vi "old code for w-on-b or b-on-w detection.vi"(9 "Numeric 2":i32, 10 "Numeric":i32, 11 "Array":sgl[](array[numeric])) -> (3 "subarray":sgl[](array[numeric]))   [LabVIEW 2011]
uses:
  <vilib>/Analysis/NI_AALBase.lvlib
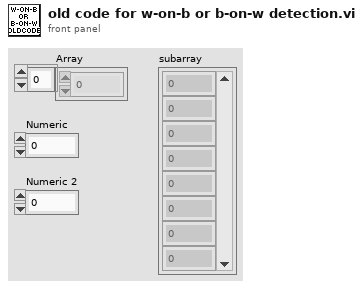
[diagram p1: front panel]
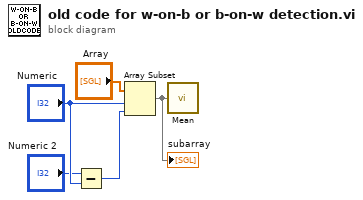
[diagram p0: block diagram]
diagram:
  n1 = Subtract(x="Numeric 2", y="Numeric") -> (x-y=w2:i32)
  n2 = Array Subset(array="Array", index="Numeric", length=w2) -> (w1:sgl[])
  "subarray" <- w1
  n3 = call <vilib>:"Mean.vi"("X"=w1) -> ()  [unwired: 2 out]
